vi "LV_PID.vi"(0 "实际位移":dbl=150.0, 2 "目标位移":dbl=150.0, 3 "PID参数":cluster{"微分系数":dbl, "积分系数":dbl, "比例系数":dbl}, 4 "正弦参数":cluster{"幅值(mm)":dbl, "中心(mm)":dbl}={"幅值(mm)"=50.0, "中心(mm)"=100.0}, 5 "方波参数":cluster{"目标位移1":dbl, "目标位移2":dbl, "占空比":dbl}={"目标位移1"=150.0, "目标位移2"=100.0, "占空比"=50.0}, 6 "输出电压上限":dbl, 7 "输出电压下限":dbl, 8 "方式":enum32{"阶跃", "正弦", "方波"}(tab)) -> (16 "输出电压":dbl, 17 "输出电压极限报警":bool)   [LabVIEW 2010]
panel:
  in  "执行次数":u32=100
  in  "采样周期":u8(knob) scale=0.0..50.0
  out "V0":dbl
  out "e3":dbl
  out "e2":dbl
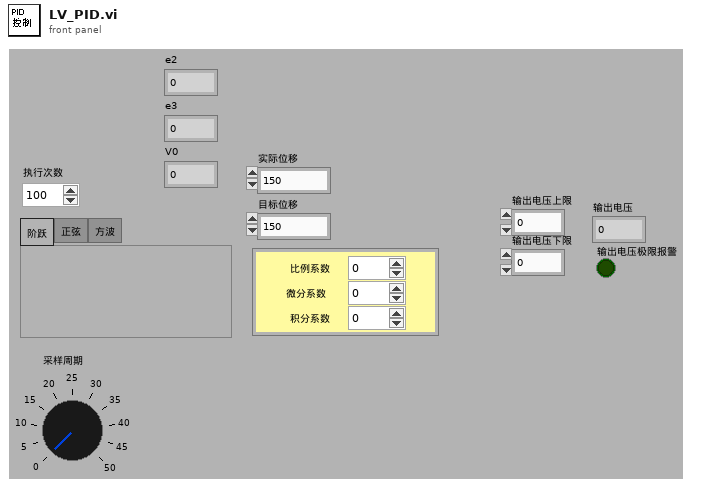
[diagram p1: front panel]
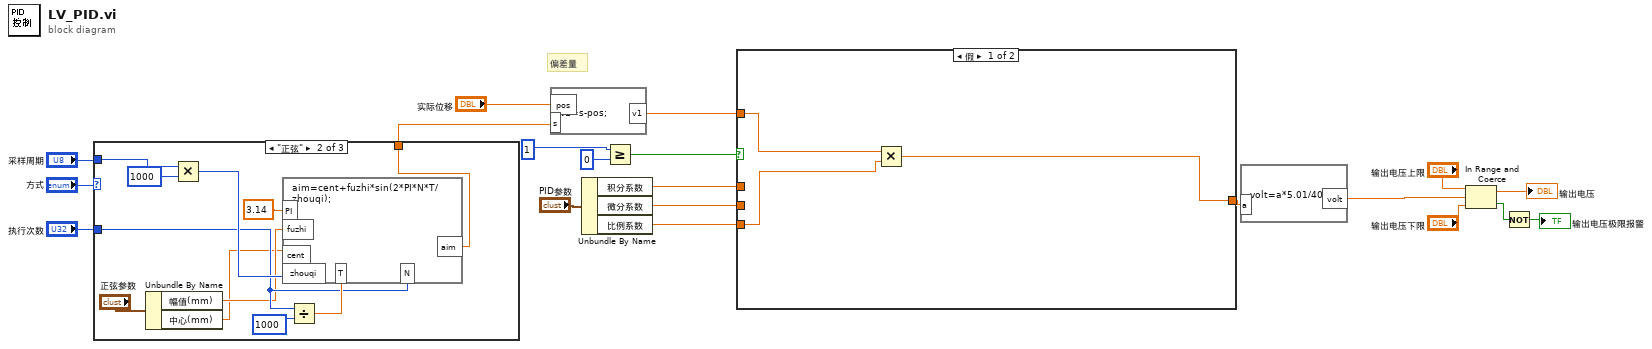
[diagram p0: block diagram]
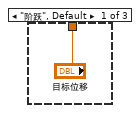
[diagram p2: hidden frame]
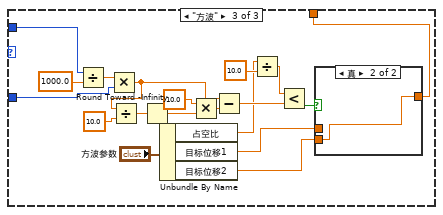
[diagram p3: hidden frame]
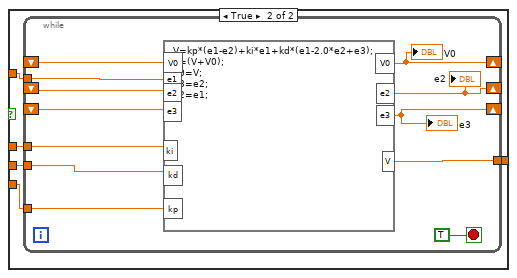
[diagram p5: hidden frame]
diagram:
  # "偏差量"
  n1 = case shown="\"正弦\"" "方式" {
    tunnel: ["目标位移" w29 w35] -> w3
    tunnel: "采样周期" -> [_ w28 w39]
    tunnel: "执行次数" -> [_ w25 w34]
    frame "阶跃", Default {
    }
    frame "正弦" {
      n2 = Unbundle By Name("正弦参数") -> ("幅值(mm)"=w23:dbl, "中心(mm)"=w22:dbl)
      n3 = Multiply(x=w28, y=u16 1000) -> (x*y=w26:u16)
      n4 = Divide(x=w25, y=u32 1000) -> (x/y=w32:dbl)
      n5 = formula code="aim=cent+fuzhi*sin(2*PI*N*T/zhouqi);"("N"=w25, "PI"=3.14 ("input variable"), "fuzhi"=w23, "cent"=w22, "zhouqi"=w26, "T"=w32) -> ("aim"=w29:dbl)
    }
    frame "方波" {
      n6 = Divide(x=w39, y=1000.0) -> (x/y=w50:dbl)
      n7 = Multiply(x=w50, y=w34) -> (x*y=w46:dbl)
      n8 = Divide(x=w46, y=10.0) -> (x/y=w45:dbl)
      n9 = Round Toward -Infinity(1:w45) -> (0:w41:dbl)
      n10 = Unbundle By Name("方波参数") -> ("占空比"=w33:dbl, "目标位移1"=w37:dbl, "目标位移2"=w36:dbl)
      n11 = Multiply(x=10.0, y=w41) -> (x*y=w43:dbl)
      n12 = Subtract(x=w46, y=w43) -> (x-y=w49:dbl)
      n13 = Divide(x=w33, y=10.0) -> (x/y=w48:dbl)
      n14 = Less?(x=w48, y=w49) -> (x < y?=w47:bool)
      n15 = case shown="真" w47 {
        tunnel: [w52 w53] -> w35
        tunnel: w37 -> [w52 _]
        tunnel: w36 -> [_ w53]
        frame False {
        }
        frame True {
        }
      }
    }
  }
  n16 = formula code="v1=s-pos;"("pos"="实际位移", "s"=w3) -> ("v1"=w17:dbl)
  n17 = Unbundle By Name("PID参数") -> ("积分系数"=w7:dbl, "微分系数"=w6:dbl, "比例系数"=w5:dbl)
  n18 = Greater Or Equal?(x=1, y=0) -> (x >= y?=w19:bool)
  n19 = case shown="假" w19 {
    tunnel: w17 -> [w56 w61]
    tunnel: [w55 w60] -> w18
    tunnel: w7 -> [_ w59]
    tunnel: w6 -> [_ w58]
    tunnel: w5 -> [w54 w57]
    frame False {
      n20 = Multiply(x=w56, y=w54) -> (x*y=w55:dbl)
    }
    frame True {
      n21 = while {
        tunnel: w61 -> [w73]
        tunnel: [w72] -> w60
        shift-right: [w69] -> _
        shift-left: _ -> [w70]
        shift-right: [w67] -> _
        shift-left: _ -> [w68]
        shift-right: [w65] -> _
        shift-left: _ -> [w66]
        tunnel: w59 -> [w64]
        tunnel: w58 -> [w63]
        tunnel: w57 -> [w62]
        stop <- TRUE stop-if-true
        n22 = formula code="V=kp*(e1-e2)+ki*e1+kd*(e1-2.0*e2+e3);\nV=(V+V0);\nV0=V;\ne3=e2;\ne2=e1;"("e1"=w73, "e2"=w66, "e3"=w68, "ki"=w64, "kd"=w63, "kp"=w62, "V0"=w70) -> ("V"=w72:dbl, "V0"=w69:dbl, "e2"=w65:dbl, "e3"=w67:dbl)
        "V0" <- w69
        "e3" <- w67
        "e2" <- w65
      }
    }
  }
  n23 = formula code="volt=a*5.01/400;"("a"=w18) -> ("volt"=w14:dbl)
  n24 = In Range and Coerce(upper limit="输出电压上限", x=w14, lower limit="输出电压下限") -> (coerced(x)=→"输出电压":dbl, In Range?=w10:bool)
  n25 = Not(x=w10) -> (.not. x?=→"输出电压极限报警":bool)
